vi "ex5.vi"() -> ()   [LabVIEW 2022 SP3]
panel:
  out "Output":string
  in  "Input":string
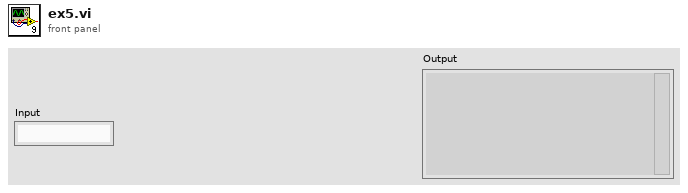
[diagram p1: front panel]
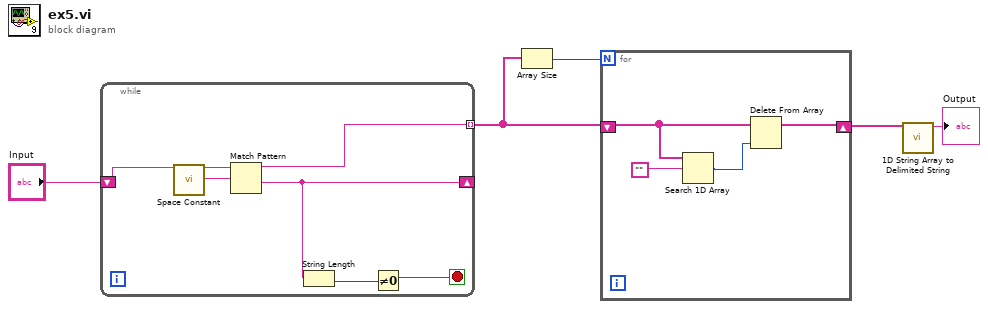
[diagram p0: block diagram]
diagram:
  n1 = while {
    shift-right: [w7] -> _
    shift-left: "Input" -> [w9]
    tunnel: [w6] -> w4 mode=indexing
    stop <- w11 stop-if-true
    n2 = call <vilib>:"Space Constant.vi"() -> ("String"=w8:string)
    n3 = Match Pattern(string=w9, regular expression=w8) -> (before substring=w6:string, after substring=w7:string)  [unwired: 1 in, 2 out]
    n4 = String Length(string=w7) -> (length=w10:i32)
    n5 = Not Equal To 0?(x=w10) -> (x != 0?=w11:bool)
  }
  n6 = Array Size(array=w4) -> (size(s)=w3:i32)
  n7 = for {
    N: w3 -> [_]
    shift-right: [w12] -> w2
    shift-left: w4 -> [w14]
    n8 = Search 1D Array(1D array=w14, element="") -> (index of element=w13:i32)  [unwired: 1 in]
    n9 = Delete From Array(array=w14, index=w13) -> (array with subset deleted=w12:string[])  [unwired: 1 in, 1 out]
  }
  n10 = call <vilib>:"1D String Array to Delimited String.vi"("string array"=w2) -> ("delimited string"=→"Output":string)  [unwired: 10 in]
